vi "AssertControlValueAlmostEqual.vi"(0 "VI Reference In":refnum<vi>, 1 "Label":string, 5 "Control Name":string, 7 "Control Value":ext, 9 "Tolerance":ext=0.00000100000000000000000004, 11 "error out":errorcluster, 12 "Timeout(5 sec)":dbl=5.0) -> (4 "VI Reference Out":refnum<vi>, 15 "error out":errorcluster)   [LabVIEW 2016]
uses:
  AssertControlValueByPathString.vi
  <vilib>/addons/_JKI Toolkits/Caraya/classes/Assert/Assert Almost Equal_Float.vi
  <vilib>/addons/_JKI Toolkits/Caraya/classes/Assert/Assert True.vi
  <vilib>/addons/_JKI Toolkits/Caraya/classes/Assert/Assert.lvclass
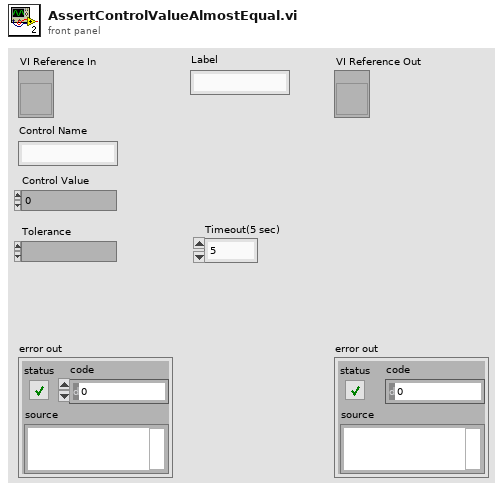
[diagram p1: front panel]
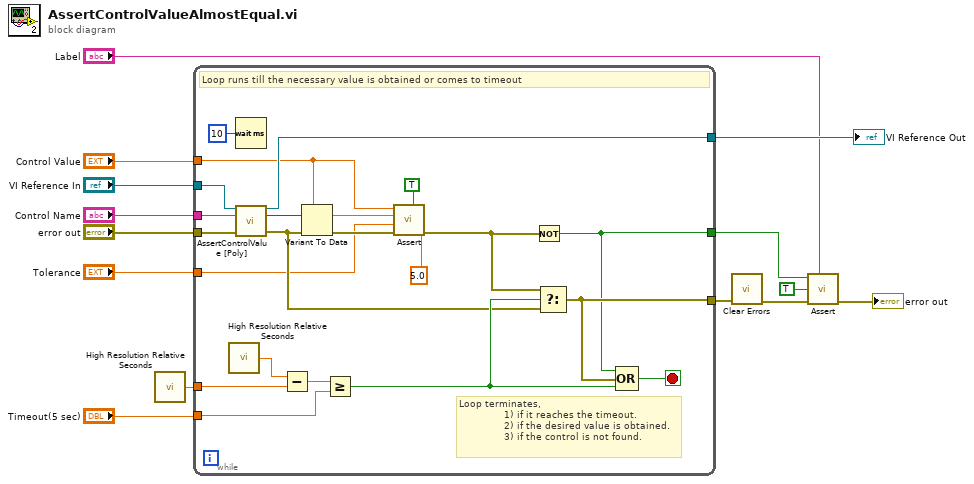
[diagram p0: block diagram]
diagram:
  n1 = call <vilib>:"High Resolution Relative Seconds.vi"() -> ("relative seconds"=w12:dbl)
  n2 = while {
    tunnel: "Control Name" -> [w35]
    tunnel: "VI Reference In" -> [w34]
    tunnel: "Control Value" -> [w23]
    tunnel: "Timeout(5 sec)" -> [w28]
    tunnel: [w31] -> w9
    tunnel: w12 -> [w33]
    tunnel: "error out" -> [w36]
    tunnel: [w24] -> w8
    tunnel: "Tolerance" -> [w18]
    tunnel: [w15] -> w4
    stop <- w27 stop-if-true
    # "Loop terminates,\n               1) if it reaches the timeout.\n               2) if the desired value is obtained.\n               3) if the control is not found."
    # "Loop runs till the necessary value is obtained or comes to timeout"
    n3 = call <vilib>:"High Resolution Relative Seconds.vi"() -> ("relative seconds"=w32:dbl)
    n4 = Wait (ms)(milliseconds to wait=u32 10) -> ()  [unwired: 1 out]
    n5 = call-poly "AssertControlValue [Poly].vi"("VI Reference In"=w34, "Control Name"=w35, "error in"=w36) -> ("VI Reference Out"=w31:refnum<vi>, "Value"=w22:variant, "error out"=w20:errorcluster)  [unwired: 10 in]
    n6 = Subtract(x=w32, y=w33) -> (x-y=w29:dbl)
    n7 = Variant To Data(error in=w20, type=w23, Variant=w22) -> (data=w21:ext, error out=w19:errorcluster)
    n8 = Greater Or Equal?(x=w29, y=w28) -> (x >= y?=w25:bool)
    n9 = call-poly <vilib>:"Assert.vi"("Execution time (s)"=5.0, "Assert Only? (F)"=TRUE, "error in (no error)"=w19, "Tolerance"=w18, "Y"=w21, "X"=w23) -> ("error out"=w26:errorcluster)  [unwired: 5 in]
    n10 = Not(x=w26) -> (.not. x?=w15:bool)
    n11 = Select(t=w26, s=w25, f=w20) -> (s? t:f=w24:errorcluster)
    n12 = Compound Arithmetic op=OR(w15, w24, w25) -> (w27:bool)
  }
  "VI Reference Out" <- w9
  n13 = call <vilib>:"Clear Errors.vi"("error in (no error)"=w8) -> ("error out"=w2:errorcluster)  [unwired: 5 in, 1 out]
  n14 = call-poly <vilib>:"Assert.vi"("Label"="Label", "error in (no error)"=w2, "Register with caller test (F)"=TRUE, "True?"=w4) -> ("error out"=→"error out":errorcluster)  [unwired: 7 in]
